vi "AutoTurnGyro.vi"(7 "Sensor (Gyro)":enum16{"Gyro", "Vision"}(ring), 8 "error in":errorcluster, 9 "Error Tolerence":dbl, 10 "Turn Amount":i32=45, 11 "Initial Angle":dbl) -> (0 "error out":errorcluster, 3 "Target Angle Out":dbl)   [LabVIEW 2012]
doc: "This VI is called when autonomous begins, and will automatically be terminated when autonomous ends. You can carry out timed or sensor driven robot movement independently without needing to return to the caller."
uses:
  <vilib>/addons/control/pid/NI_PID_pid.lvlib
  <vilib>/addons/control/pid/pid.llb/PID (DBL).vi
  Robot Global Data.vi
  <vilib>/Rock Robotics/WPI/RobotDrive/WPI_RobotDriveArcadeDrive_Standard(NoSaturation).vi
panel:
  in  "PID gains":T1={"proportional gain (Kc)"=1.0, "integral time (Ti, min)"=0.0, "derivative time (Td, min)"=0.0}
  out "Graph":cluster{dbl, "output":dbl}(graph)
  out "PID Output":dbl format="%.2f"
  out "Error":dbl
  out "Current Angle":dbl
  # "Low gear\nMax turn - 0.71\nMin turn - 0.45"
  # "P: 1"
  # "Curve Value Input Not used when using Gyro"
  # "\"-\" Turns Left\n\"+\" Turns Right"
  # "If Using Gyro:\nEnter Turn amount in Degrees:\n\"-\" AngleTurns Left\n\"+\" Angle Turns Right"
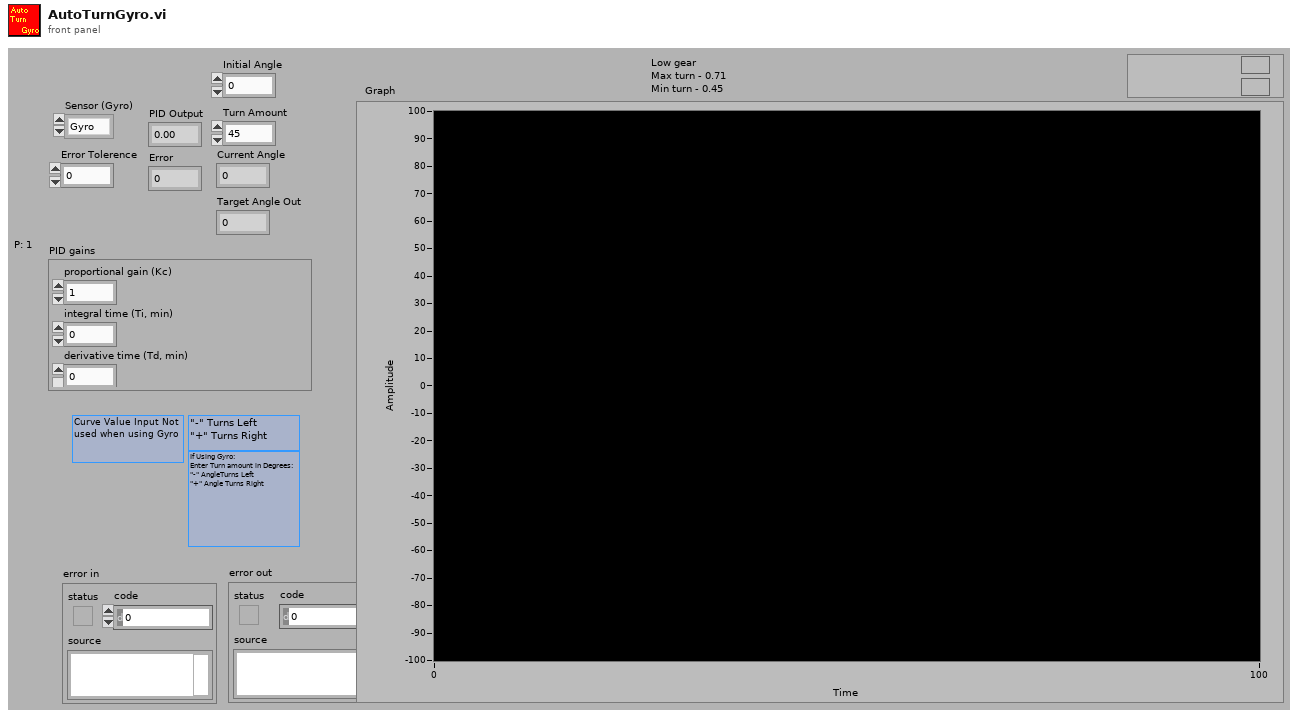
[diagram p1: front panel]
types:
  T1 = cluster{"proportional gain (Kc)":dbl, "integral time (Ti, min)":dbl, "derivative time (Td, min)":dbl}
  T2 = typedef "WPI_GyroDevRef.ctl" = cluster{"DevStatus":errorcluster, "Analog Module":T3, "Analog Channel":T4, "Offset":dbl, "Gain (VoltsPerDegree/Second)":dbl}
  T3 = typedef "FPGA_TypedefAnalogModule.ctl" = enum16{"Analog Module 1", "Analog Module 2"}
  T4 = typedef "FPGA_AIChannel.ctl" = enum8{"AI 1", "AI 2", "AI 3", "AI 4", "AI 5", "AI 6", "AI 7", "AI 8", "Invalid"}
  T5 = typedef "WPI_RobotDriveDevRef.ctl" = cluster{"DevStatus":errorcluster, "Motors[]":T6[], "Square Inputs":bool, "Max Output":dbl, "Isochronous":bool}
  T6 = typedef "WPI_MotorControlDeviceRef.ctl" = cluster{"DeviceStatus":errorcluster, "Type":enum16{"PWM", "CAN"}, "PWM":cluster{"Digital Module":T7, "PWM Channel":T8, "DeadBand":T9}, "CAN":cluster{"Device Number":u8, "Control Mode":T10, "Semaphore":T11, "Max Vout":dbl}, "Invert":bool, "TransformRef":T12, "InvTransformRef":T12}
  T7 = typedef "FPGA_TypedefDigitalModule.ctl" = enum16{"Digital Module 1", "Digital Module 2"}
  T8 = typedef "FPGA_DIOPWMChannel.ctl" = enum8{"PWM 1", "PWM 2", "PWM 3", "PWM 4", "PWM 5", "PWM 6", "PWM 7", "PWM 8", "PWM 9", "PWM 10", "Invalid"}
  T9 = typedef "WPI_PWMDeadband.ctl" = cluster{"Name":string, "maxPositivePwm":i32, "minPositivePwm":i32, "centerPwm":i32, "maxNegativePwm":i32, "minNegativePwm":i32, "angularRange":u16}
  T10 = typedef "WPI_CANJaguar_ControlMode.ctl" = enum8{"Percent VBus", "Current", "Speed", "Position", "Voltage"}
  T11 = typedef "Semaphore RefNum" = refnum<k1>
  T12 = typedef "WPI_PWMTransform_ConPane.ctl" = refnum<vi>
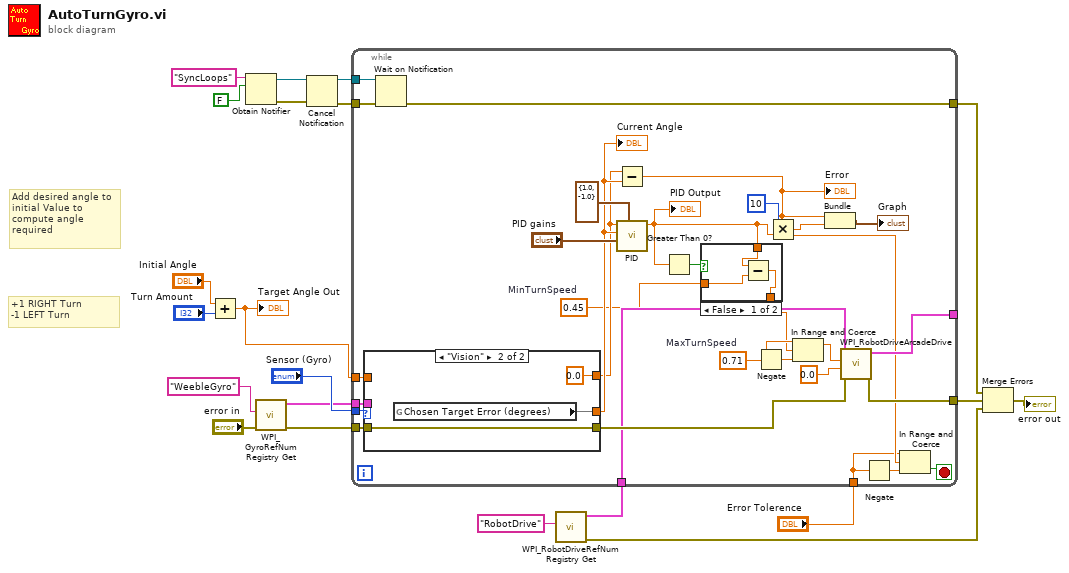
[diagram p0: block diagram]
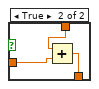
[diagram p2: hidden frame]
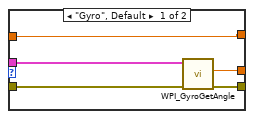
[diagram p3: hidden frame]
diagram:
  # "+1 RIGHT Turn\n-1 LEFT Turn"
  # "Add desired angle to initial Value to\ncompute angle required"
  n1 = Add(x="Initial Angle", y="Turn Amount") -> (x+y=w8:dbl)
  "Target Angle Out" <- w8
  n2 = Obtain Notifier(name (unnamed)="SyncLoops", notification data type=FALSE) -> (notifier out=w4:refnum<notifier>, error out=w2:errorcluster)  [unwired: 2 in, 1 out]
  n3 = call <vilib>:"WPI_GyroRefNum Registry Get.vi"("error in (no error)"="error in", "refnum name"="WeebleGyro") -> ("error out"=w12:errorcluster, "GyroDevRef"=w13:T2)  [unwired: 8 in]
  n4 = Cancel Notification(0:w4, 3:w2) -> (8:w5:refnum<notifier>, 11:w3:errorcluster)  [unwired: 1 out]
  n5 = call <vilib>:"WPI_RobotDriveRefNum Registry Get.vi"("refnum name"="RobotDrive") -> ("error out"=w9:errorcluster, "RobotDriveDevRef"=w11:T5)  [unwired: 9 in]
  n6 = while {
    tunnel: [w51] -> _
    tunnel: [w46] -> w10
    tunnel: "Sensor (Gyro)" -> [w44]
    tunnel: "Error Tolerence" -> [w41]
    tunnel: w13 -> [w40]
    tunnel: w12 -> [w38]
    tunnel: w11 -> [w37]
    tunnel: w8 -> [w36]
    tunnel: w5 -> [w24]
    tunnel: w3 -> [w23]
    tunnel: [w22] -> w1
    stop <- w50 stop-if-true
    w31 = 0.71  # MaxTurnSpeed
    w28 = 0.45  # MinTurnSpeed
    n7 = case shown="\"Vision\"" w44 {
      tunnel: [w62 w64] -> w47
      tunnel: w40 -> [w61 _]
      tunnel: [w59 w65] -> w39
      tunnel: w38 -> [w60 w65]
      tunnel: w36 -> [w58 _]
      tunnel: [w58 0.0] -> w35
      frame "Gyro", Default {
        n8 = call <vilib>:"WPI_GyroGetAngle.vi"("error in (no error)"=w60, "GyroDevRef"=w61) -> ("error out"=w59:errorcluster, "Angle"=w62:dbl)  [unwired: 8 out]
      }
      frame "Vision" {
        n9 = global read "Robot Global Data.vi" "Chosen Target Error (degrees)"() -> (w64)
      }
    }
    "Current Angle" <- w47
    n10 = Wait on Notification(notifier=w24, error in (no error)=w23) -> (error out=w22:errorcluster)  [unwired: 2 in, 3 out]
    n11 = Subtract(x=w35, y=w47) -> (x-y=w43:dbl)
    "Error" <- w43
    n12 = call-poly <vilib>:"PID.vi"("output range"=cluster{"output high":dbl, "output low":dbl} {"output high"=1.0, "output low"=-1.0}, "PID gains"="PID gains", "process variable"=w47, "setpoint"=w35) -> ("output"=w26:dbl)  [unwired: 2 in, 5 out]
    "PID Output" <- w26
    n13 = Greater Than 0?(x=w26) -> (x > 0?=w29:bool)
    n14 = case shown="False" w29 {
      tunnel: [w53 w57] -> w30
      tunnel: w26 -> [w54 w56]
      tunnel: w28 -> [w52 w55]
      frame False {
        n15 = Subtract(x=w54, y=w52) -> (x-y=w53:dbl)
      }
      frame True {
        n16 = Add(x=w56, y=w55) -> (x+y=w57:dbl)
      }
    }
    n17 = Negate(x=w31) -> (-x=w32:dbl)
    n18 = Multiply(x=10, y=w26) -> (x*y=w27:dbl)
    n19 = In Range and Coerce(upper limit=w31, x=w30, lower limit=w32) -> (coerced(x)=w33:dbl)  [unwired: 1 out]
    n20 = Bundle(w43, w27) -> (→"Graph":cluster{dbl, dbl})  [unwired: 1 out]
    n21 = call-poly <vilib>:"WPI_RobotDriveArcadeDrive.vi"("error in (no error)"=w39, "Y axis value"=0.0, "X axis value"=w33, "RobotDriveDevRef"=w37) -> ("error out"=w46:errorcluster, "RobotDriveDevRef"=w51:T5)  [unwired: 5 in, 1 out]
    n22 = Negate(x=w41) -> (-x=w42:dbl)
    n23 = In Range and Coerce(upper limit=w41, x=w43, lower limit=w42) -> (In Range?=w50:bool)  [unwired: 1 out]
  }
  n24 = Merge Errors(w1, w10, w9) -> (→"error out":errorcluster)
